vi "Set Objective.vi"(0 "Notifier Name In":string, 2 "Wait for Finish":bool=TRUE, 7 "Objective Index":u8, 11 "Error In":errorcluster) -> (4 "Notifier Name Out":string, 15 "Error Out":errorcluster)   [LabVIEW 2020]
uses:
  Microscopes Type Defs/Microscope Notifier.ctl
  Microscopes Type Defs/Microscope Actions.ctl
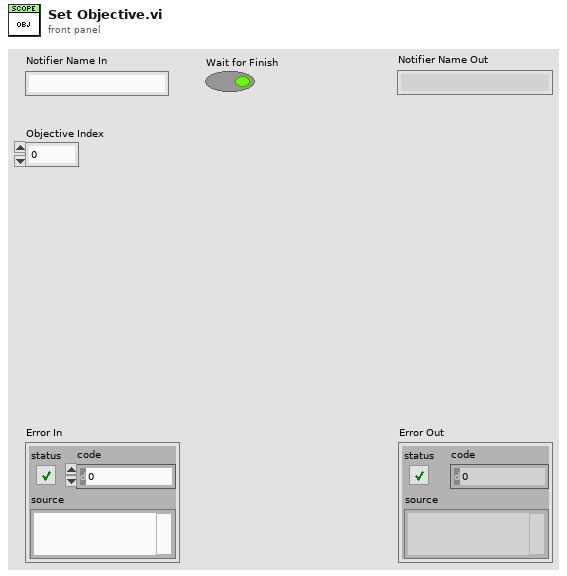
[diagram p1: front panel]
types:
  T1 = typedef "Microscope Notifier.ctl" = cluster{"Actions":T2, "Action Done":bool, "Objective Index":u8, "Objective Z Position (um)":dbl, "Lamp Index":u8, "Lamp State":bool, "Output Port":u8, "Shutter Index":u8, "Shutter State":bool, "Dichroic Wheel Position":u8, "Parameter":string, "Parameter Value":string, "Base Locked?":bool, "Obj Speed":u32, "Obj Acceleration":u32, "Obj Deceleration":u32, "Lamp Power (%)":dbl}
  T2 = typedef "Microscope Actions.ctl" = enum16{"Do Nothing", "Lock Base", "Lock Focus Knob", "Get Objective Index", "Get Objective Z Position", "Get Lamp State", "Get Lamp Power", "Get Output Port", "Get Shutter State", "Get Dichroic Wheel Position", "Set Lamp Index", "Set Shutter Index", "Set Objective Z Position", "Set Lamp State", "Set Lamp Power", "Set Output Port", "Set Shutter State", "Set Dichroic Wheel Position", "Set Objective", "Abort Move", "Set Parameter", "Get Parameter", "Quit"}
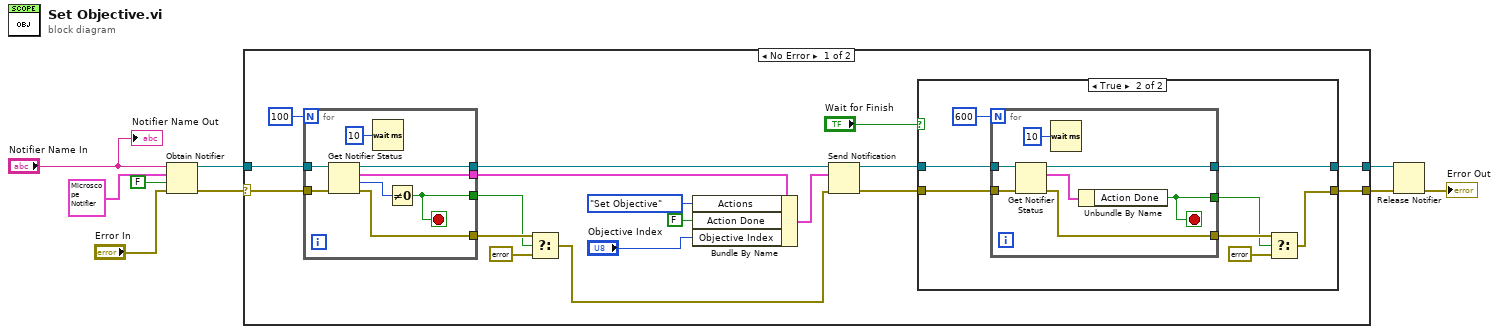
[diagram p0: block diagram]
diagram:
  n1 = Obtain Notifier(name (unnamed)="Notifier Name In", notification data type=T1 {"Actions"=enum."Get Objective Index", "Action Done"=FALSE, "Objective Index"=0, "Objective Z Position (um)"=0.0, "Lamp Index"=0, "Lamp State"=FALSE, "Output Port"=0, "Shutter Index"=0, "Shutter State"=FALSE, "Dichroic Wheel Position"=0, "Parameter"="", "Parameter Value"="", "Base Locked?"=FALSE, "Obj Speed"=0, "Obj Acceleration"=0, "Obj Deceleration"=0, "Lamp Power (%)"=0.0} ("Microscope Notifier"), create if not found? (T)=FALSE, error in (no error)="Error In") -> (notifier out=w6:refnum<notifier>, error out=w7:errorcluster)  [unwired: 1 out]
  n2 = case shown="No Error" w7 {
    selector: w7 -> [w25 w54]
    tunnel: w6 -> [w27 w53]
    tunnel: [w16 w54] -> w2
    tunnel: [w17 w53] -> w3
    frame No Error {
      n3 = for {
        N: 100 -> [_]
        tunnel: w27 -> [w52]
        tunnel: [w50] -> w13
        tunnel: [w48] -> w23
        tunnel: w25 -> [w47]
        tunnel: [w46] -> w14
        tunnel: [w45] -> w24
        stop <- w50 stop-if-true
        n4 = Get Notifier Status(notifier=w52, error in (no error)=w47) -> (notifier out=w48:refnum<notifier>, current notification=w45:T1, # waiting=w51:i32, error out=w46:errorcluster)  [unwired: 1 out]
        n5 = Wait (ms)(milliseconds to wait=u32 10) -> ()  [unwired: 1 out]
        n6 = Not Equal To 0?(x=w51) -> (x != 0?=w50:bool)
      }
      n7 = Select(t=w14, s=w13, f=errorcluster {"status"=TRUE, "code"=0, "source"="IX81 Base Error: Base busy time out."}) -> (s? t:f=w10:errorcluster)
      n8 = Bundle By Name(cluster=w24, "Actions"=Microscope_Actions."Set Objective", "Action Done"=FALSE, "Objective Index"="Objective Index") -> (w22:T1)
      n9 = Send Notification(notification=w22, notifier=w23, error in (no error)=w10) -> (notifier out=w18:refnum<notifier>, error out=w21:errorcluster)
      n10 = case shown="True" "Wait for Finish" {
        tunnel: w21 -> [w28 w37]
        tunnel: w18 -> [w29 w36]
        tunnel: [w29 w35] -> w17
        tunnel: [w28 w34] -> w16
        frame False {
        }
        frame True {
          n11 = for {
            N: 600 -> [_]
            tunnel: w36 -> [w44]
            tunnel: [w42] -> w35
            tunnel: w37 -> [w41]
            tunnel: [w40] -> w32
            tunnel: [w38] -> w31
            stop <- w38 stop-if-true
            n12 = Get Notifier Status(notifier=w44, error in (no error)=w41) -> (notifier out=w42:refnum<notifier>, current notification=w39:T1, error out=w40:errorcluster)  [unwired: 2 out]
            n13 = Wait (ms)(milliseconds to wait=u32 10) -> ()  [unwired: 1 out]
            n14 = Unbundle By Name(w39) -> ("Action Done"=w38:bool)
          }
          n15 = Select(t=w32, s=w31, f=errorcluster {"status"=TRUE, "code"=0, "source"="IX81 Base Error: Action didn't complete."}) -> (s? t:f=w34:errorcluster)
        }
      }
    }
    frame Error {
    }
  }
  n16 = Release Notifier(notifier=w3, error in (no error)=w2) -> (error out=→"Error Out":errorcluster)  [unwired: 1 in, 2 out]
  "Notifier Name Out" <- "Notifier Name In"
